vi "Vision Processing.vi"(4 "error in (no error)":errorcluster, 7 "Image Size":T1=enum."320x240") -> ()   [LabVIEW 2017]
doc: "This VI runs in parallel to other tasks. It gets images from the camera, processes them for color or shape and uses commands or globals to affect the behavior of other subsystems."
uses:
  <vilib>/Rock Robotics/WPI/Camera/WPI_CameraImageSize.ctl
  <vilib>/Rock Robotics/WPI/Camera/WPI_CameraWhite Balance Values.ctl
  <vilib>/Rock Robotics/WPI/Camera/WPI_CameraExposure Values.ctl
  <vilib>/Rock Robotics/WPI/Camera/WPI_CameraFrameRate.ctl
  Framework/Robot Global Data.vi
panel:
  in  "Image Size 2":T1=enum."320x240"
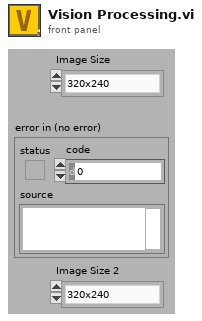
[diagram p1: front panel]
types:
  T1 = typedef "WPI_CameraImageSize.ctl" = enum16{"640x480", "320x240", "160x120", "Custom"}
  T2 = typedef "WPI_CameraFrameRate.ctl" = u32
  T3 = typedef "WPI_CameraExposure Values.ctl" = enum16{"Auto", "Flicker-free 50 Hz", "Flicker-free 60 Hz", "Hold current", "Custom"}
  T4 = typedef "WPI_CameraWhite Balance Values.ctl" = enum16{"Auto", "Fixed indoor", "Fixed outdoor 1", "Fixed outdoor 2", "Fixed fluorescent 1", "Fixed fluorescent 2", "Hold current", "Custom"}
  T5 = typedef "Image Type" = u32
  T6 = typedef "WPI_CameraDevRef.ctl" = cluster{"Camera Address":string, "CameraStatus":errorcluster}
  T7 = typedef "IMAQ Image.ctl" = refnum<image>
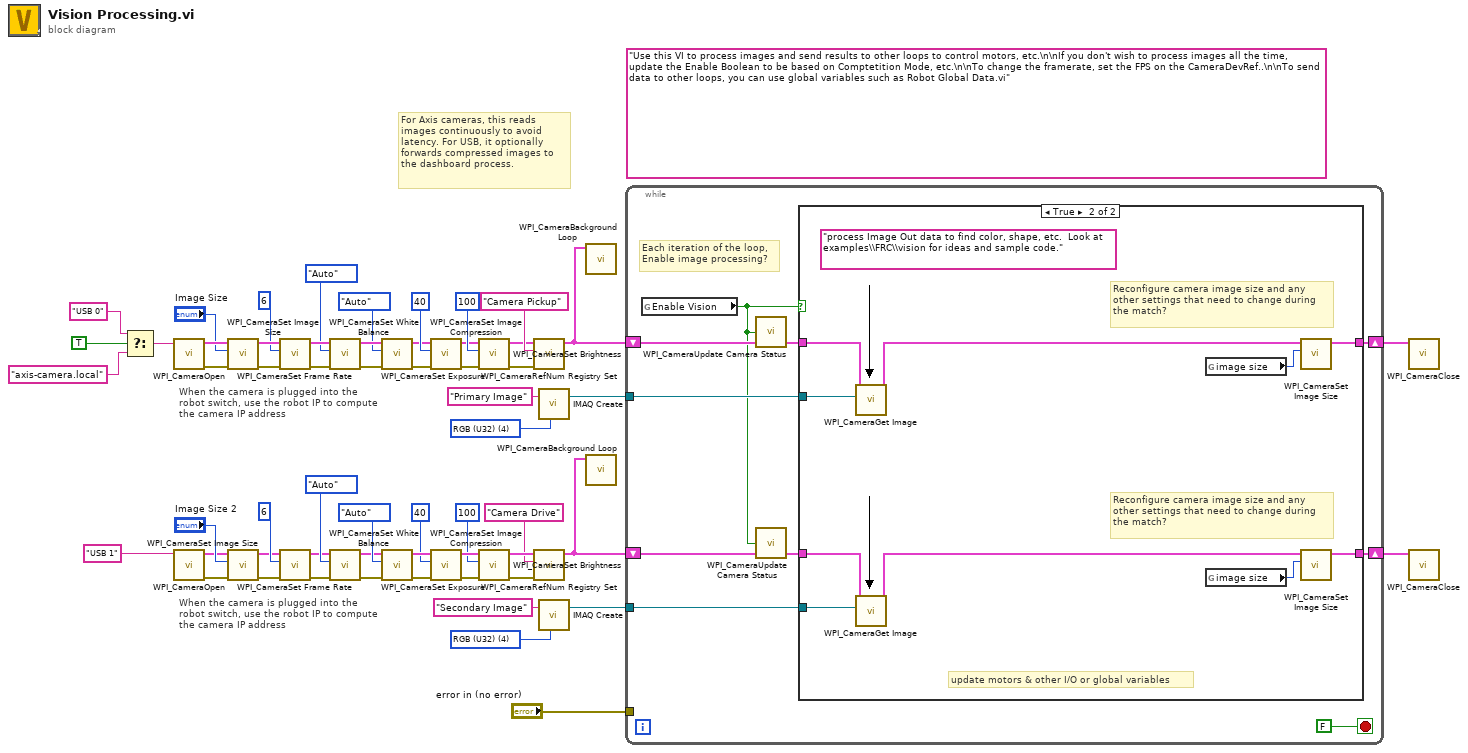
[diagram p0: block diagram]
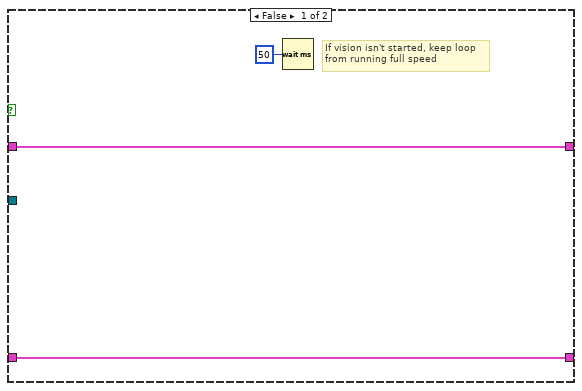
[diagram p2: hidden frame]
diagram:
  w5 = T5 4 items=["Grayscale (U8)", "Grayscale (I16)", "Grayscale (SGL)", "Complex (CSG)", "RGB (U32)", "HSL (U32)", "RGB (U64)"] ("Image Type")
  (unwired) "Use this VI to process images and send results to other loops to control motors, etc.\n\nIf you don't wish to process images all the time, update the Enable Boolean to be based on Comptetition Mode, etc.\n\nTo change the framerate, set the FPS on the CameraDevRef..\n\nTo send data to other loops, you can use global variables such as Robot Global Data.vi"
  w58 = T5 4 items=["Grayscale (U8)", "Grayscale (I16)", "Grayscale (SGL)", "Complex (CSG)", "RGB (U32)", "HSL (U32)", "RGB (U64)"] ("Image Type")
  # "When the camera is plugged into the\nrobot switch, use the robot IP to compute\nthe camera IP address"
  # "When the camera is plugged into the\nrobot switch, use the robot IP to compute\nthe camera IP address"
  # "For Axis cameras, this reads\nimages continuously to avoid\nlatency. For USB, it optionally\nforwards compressed images to\nthe dashboard process."
  n1 = Select(t="USB 0" ("format string"), s=TRUE ("dot notation? (F)"), f="axis-camera.local" ("format string")) -> (s? t:f=w29:string)
  n2 = call <vilib>:"WPI_CameraOpen.vi"("Camera Address"=w29) -> ("error out"=w46:errorcluster, "CameraDevRef"=w47:T6)  [unwired: 1 in, 8 out]
  n3 = call <vilib>:"WPI_CameraOpen.vi"("Camera Address"="USB 1" ("format string")) -> ("error out"=w16:errorcluster, "CameraDevRef"=w15:T6)  [unwired: 1 in, 8 out]
  n4 = call <vilib>:"WPI_CameraSet Image Size.vi"("error in (no error)"=w46, "Image Size"="Image Size", "CameraDevRef"=w47) -> ("error out"=w45:errorcluster, "CameraDevRef Out"=w48:T6)  [unwired: 1 in, 6 out]
  n5 = call <vilib>:"WPI_CameraSet Image Size.vi"("error in (no error)"=w16, "Image Size"="Image Size 2", "CameraDevRef"=w15) -> ("error out"=w17:errorcluster, "CameraDevRef Out"=w14:T6)  [unwired: 1 in, 6 out]
  n6 = call <vilib>:"WPI_CameraSet Frame Rate.vi"("error in (no error)"=w45, "Frame Rate (fps)"=T2 6, "CameraDevRef"=w48) -> ("error out"=w44:errorcluster, "CameraDevRef Out"=w50:T6)  [unwired: 7 out]
  n7 = call <vilib>:"WPI_CameraSet Frame Rate.vi"("error in (no error)"=w17, "Frame Rate (fps)"=T2 6, "CameraDevRef"=w14) -> ("error out"=w18:errorcluster, "CameraDevRef Out"=w12:T6)  [unwired: 7 out]
  n8 = call <vilib>:"WPI_CameraSet White Balance.vi"("error in (no error)"=w44, "White Balance"=WPI_CameraWhite_Balance_Values."Auto", "CameraDevRef"=w50) -> ("error out"=w43:errorcluster, "CameraDevRef Out"=w49:T6)  [unwired: 1 in, 6 out]
  n9 = call <vilib>:"WPI_CameraSet White Balance.vi"("error in (no error)"=w18, "White Balance"=WPI_CameraWhite_Balance_Values."Auto", "CameraDevRef"=w12) -> ("error out"=w19:errorcluster, "CameraDevRef Out"=w13:T6)  [unwired: 1 in, 6 out]
  n10 = call <vilib>:"WPI_CameraSet Exposure.vi"("error in (no error)"=w43, "Exposure"=WPI_CameraExposure_Values."Auto", "CameraDevRef"=w49) -> ("error out"=w42:errorcluster, "CameraDevRef Out"=w52:T6)  [unwired: 1 in, 6 out]
  n11 = call <vilib>:"WPI_CameraSet Exposure.vi"("error in (no error)"=w19, "Exposure"=WPI_CameraExposure_Values."Auto", "CameraDevRef"=w13) -> ("error out"=w20:errorcluster, "CameraDevRef Out"=w10:T6)  [unwired: 1 in, 6 out]
  n12 = call <vilib>:"WPI_CameraSet Image Compression.vi"("error in (no error)"=w42, "Compression"=40, "CameraDevRef"=w52) -> ("error out"=w41:errorcluster, "CameraDevRef Out"=w51:T6)  [unwired: 7 out]
  n13 = call <vilib>:"WPI_CameraSet Image Compression.vi"("error in (no error)"=w20, "Compression"=40, "CameraDevRef"=w10) -> ("error out"=w21:errorcluster, "CameraDevRef Out"=w11:T6)  [unwired: 7 out]
  n14 = call <vilib>:"WPI_CameraSet Brightness.vi"("error in (no error)"=w41, "Brightness"=100, "CameraDevRef"=w51) -> ("error out"=w39:errorcluster, "CameraDevRef Out"=w40:T6)  [unwired: 1 in, 6 out]
  n15 = call <vilib>:"WPI_CameraSet Brightness.vi"("error in (no error)"=w21, "Brightness"=100, "CameraDevRef"=w11) -> ("error out"=w23:errorcluster, "CameraDevRef Out"=w22:T6)  [unwired: 1 in, 6 out]
  n16 = call <vilib>:"WPI_CameraRefNum Registry Set.vi"("error in (no error)"=w39, "refnum name"="Camera Pickup", "CameraDevRef"=w40) -> ("CameraDevRef"=w35:T6)  [unwired: 1 in, 7 out]
  n17 = call <vilib>:"WPI_CameraRefNum Registry Set.vi"("error in (no error)"=w23, "refnum name"="Camera Drive", "CameraDevRef"=w22) -> ("CameraDevRef"=w3:T6)  [unwired: 1 in, 7 out]
  n18 = call "IMAQ Create"("Image Name"="Primary Image", "Image Type"=w58) -> ("New Image"=w56:T7)  [unwired: 2 in, 2 out]
  n19 = call "IMAQ Create"("Image Name"="Secondary Image", "Image Type"=w5) -> ("New Image"=w2:T7)  [unwired: 2 in, 2 out]
  n20 = call <vilib>:"WPI_CameraBackground Loop.vi"("CameraDevRef"=w35) -> ()  [unwired: 11 in]
  n21 = call <vilib>:"WPI_CameraBackground Loop.vi"("CameraDevRef"=w3) -> ()  [unwired: 11 in]
  n22 = while {
    shift-right: [w67] -> w33
    shift-left: w35 -> [w65]
    tunnel: w56 -> [w66]
    tunnel: "error in (no error)" -> [_]
    shift-right: [w61] -> w4
    shift-left: w3 -> [w62]
    tunnel: w2 -> [w60]
    stop <- FALSE stop-if-true
    # "Each iteration of the loop,\nEnable image processing?"
    n23 = global read "Robot Global Data.vi" "Enable Vision"() -> (w59:bool)
    n24 = call <vilib>:"WPI_CameraUpdate Camera Status.vi"("CameraDevRef In"=w65, "Enable Vision"=w59) -> ("CameraDevRef Out"=w64:T6)  [unwired: 3 in]
    n25 = call <vilib>:"WPI_CameraUpdate Camera Status.vi"("CameraDevRef In"=w62, "Enable Vision"=w59) -> ("CameraDevRef Out"=w63:T6)  [unwired: 3 in]
    n26 = case shown="True" w59 {
      tunnel: w66 -> [_ w80]
      tunnel: [w71 w81] -> w67
      tunnel: w64 -> [w71 w78]
      tunnel: w60 -> [_ w73]
      tunnel: [w69 w72] -> w61
      tunnel: w63 -> [w69 w75]
      frame False {
        # "If vision isn't started, keep loop\nfrom running full speed"
        n27 = Wait (ms)(milliseconds to wait=u32 50) -> ()  [unwired: 1 out]
      }
      frame True {
        (unwired) "process Image Out data to find color, shape, etc.  Look at examples\\FRC\\vision for ideas and sample code."
        # "Reconfigure camera image size and any\nother settings that need to change during\nthe match?"
        # "update motors & other I/O or global variables"
        # "Reconfigure camera image size and any\nother settings that need to change during\nthe match?"
        n28 = call <vilib>:"WPI_CameraGet Image.vi"("Image"=w80, "CameraDevRef"=w78) -> ("CameraDevRef Out"=w77:T6)  [unwired: 1 in, 8 out]
        n29 = call <vilib>:"WPI_CameraGet Image.vi"("Image"=w73, "CameraDevRef"=w75) -> ("CameraDevRef Out"=w76:T6)  [unwired: 1 in, 8 out]
        n30 = global read "Robot Global Data.vi" "image size"() -> (w79:T1)
        n31 = global read "Robot Global Data.vi" "image size"() -> (w74:T1)
        n32 = call <vilib>:"WPI_CameraSet Image Size.vi"("Image Size"=w79, "CameraDevRef"=w77) -> ("CameraDevRef Out"=w81:T6)  [unwired: 2 in, 7 out]
        n33 = call <vilib>:"WPI_CameraSet Image Size.vi"("Image Size"=w74, "CameraDevRef"=w76) -> ("CameraDevRef Out"=w72:T6)  [unwired: 2 in, 7 out]
      }
    }
  }
  n34 = call <vilib>:"WPI_CameraClose.vi"("CameraDevRef"=w33) -> ()  [unwired: 1 in, 10 out]
  n35 = call <vilib>:"WPI_CameraClose.vi"("CameraDevRef"=w4) -> ()  [unwired: 1 in, 10 out]
